vi "Main.vi"(9 "Micro":string, 10 "VISA Com Port":refnum<visa-resource-name>, 11 "Module Admin":refnum<class "Delacor_lib_QMH_Cloneable Module Admin.lvclass">) -> ()   [LabVIEW 2020, in "Serial Device.lvlib"]
doc: "This template is based off of the Queued Message Handler design pattern and the Queued Message Handler project template that ships with LabVIEW.\n\nThe main difference is that the queue is private to this module and communication between modules is performed via Broadcast and Request events.\n\nRequest events are wrapped in public API methods and are handled in the Event Handling Loop (EHL) of this VI. Any module can register for Broadcast events sent by this module. The EHL generates messages based on user interface actions.\n\nThe Message Handling Loop (MHL) processes messages generated by the EHL, or by other messages. The messages are string values, so new messages can be added easily to the Message Cases case structure in the MHL. Each message cluster can also provide an optional value for Message Data, which is a variant that can be converted to whatever message-specific data is required.\n_____\nBased on Delacor QMH Project Template 5.0.0.82."
uses:
  Serial Device.lvlib
  Module Data--cluster.ctl
  <vilib>/Delacor/Delacor QMH/Libraries/Message Queue_class/Delacor_lib_QMH_Message Queue.lvclass
  <vilib>/Delacor/Delacor QMH/Libraries/Message Queue_class/Delacor_lib_QMH_Enqueue Message (Single).vi
  <vilib>/ErrorRing/Error Ring.xnode
  <vilib>/Utility/error.llb/Error Cluster From Error Code.vi
  <vilib>/Delacor/Delacor QMH/Libraries/Cloneable Module Admin_class/Delacor_lib_QMH_Cloneable Module Admin.lvclass
  Stop Argument--cluster.ctl
  <vilib>/Utility/miscctls.llb/LVPointTypeDef.ctl
  Write Port (Reply Payload)--cluster.ctl
  Write Port Argument--cluster.ctl
  Abstract/Serial Device/Serial Device.lvclass
  Implementation/Simulado/Simulado.lvclass
  Implementation/NXP/NXP.lvclass
  Implementation/Cypress/Cypress.lvclass
  C:/Users/celun/Desktop/FORK/ProyectoFinalIV2020/LectorADC3Micros/Abstract/Serial Device/Serial Device.lvclass
  C:/Users/celun/Desktop/FORK/ProyectoFinalIV2020/LectorADC3Micros/Implementation/Simulado/Simulado.lvclass
  C:/Users/celun/Desktop/FORK/ProyectoFinalIV2020/LectorADC3Micros/Implementation/NXP/NXP.lvclass
  C:/Users/celun/Desktop/FORK/ProyectoFinalIV2020/LectorADC3Micros/Implementation/Cypress/Cypress.lvclass
panel:
  out "Response":string
  in  "Read ADC":bool
  in  "ADC Channel":dbl
  in  "Set Value":bool
  in  "OFF/ON":bool
  in  "Pín":dbl
  in  "Port 2":dbl
  in  "Read Pin":bool
  out "Value":bool
  in  "Pín 2":dbl
  in  "Port 3":dbl
  in  "Set Port":bool
  in  "Value":string
  in  "Port":dbl
  out "Leds":bool[](array[boolean])
  in  "Read Pin 2":bool
  in  "Port 4":dbl
  out "error out":errorcluster
  out "Status":string
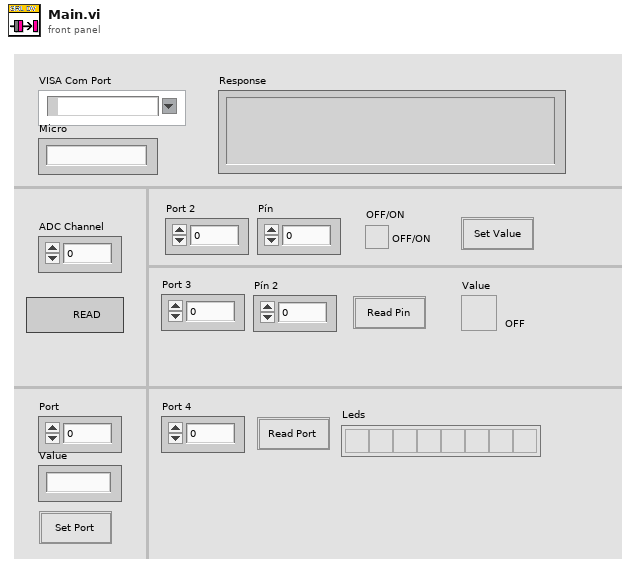
[diagram p1: front panel]
types:
  T1 = typedef "Serial Device.lvlib/Request Events--cluster.ctl" = cluster{"Stop Module":refnum<user-event>, "Show Panel":refnum<user-event>, "Hide Panel":refnum<user-event>, "Show Diagram":refnum<user-event>, "Get Module Execution Status":refnum<user-event>, "Write Port":refnum<user-event>}
  T2 = typedef "Serial Device.lvlib/Module Data--cluster.ctl" = cluster{"Status":string}
  T3 = enum32{"invalid lock state", "Not Locked", "Locked (No Password)", "Password-protected"}
  T4 = typedef "Serial Device.lvlib/Stop Argument--cluster.ctl" = cluster{"Module ID":i32, "Origin":string, "Exit via Stop Module Req?":bool, "Wait for Module to stop?":bool}
  T5 = typedef "Serial Device.lvlib/Write Port Argument--cluster.ctl" = cluster{"Module ID":i32, "Value":string, "Port":dbl, "Wait Notifier":refnum<notifier>, "wait for reply":bool}
  T6 = enum32{"Invalid", "Standard", "Closed", "Hidden", "Minimized", "Maximized"}
  T7 = typedef "LVPointTypeDef.ctl" = cluster{"Horizontal":i16, "Vertical":i16}
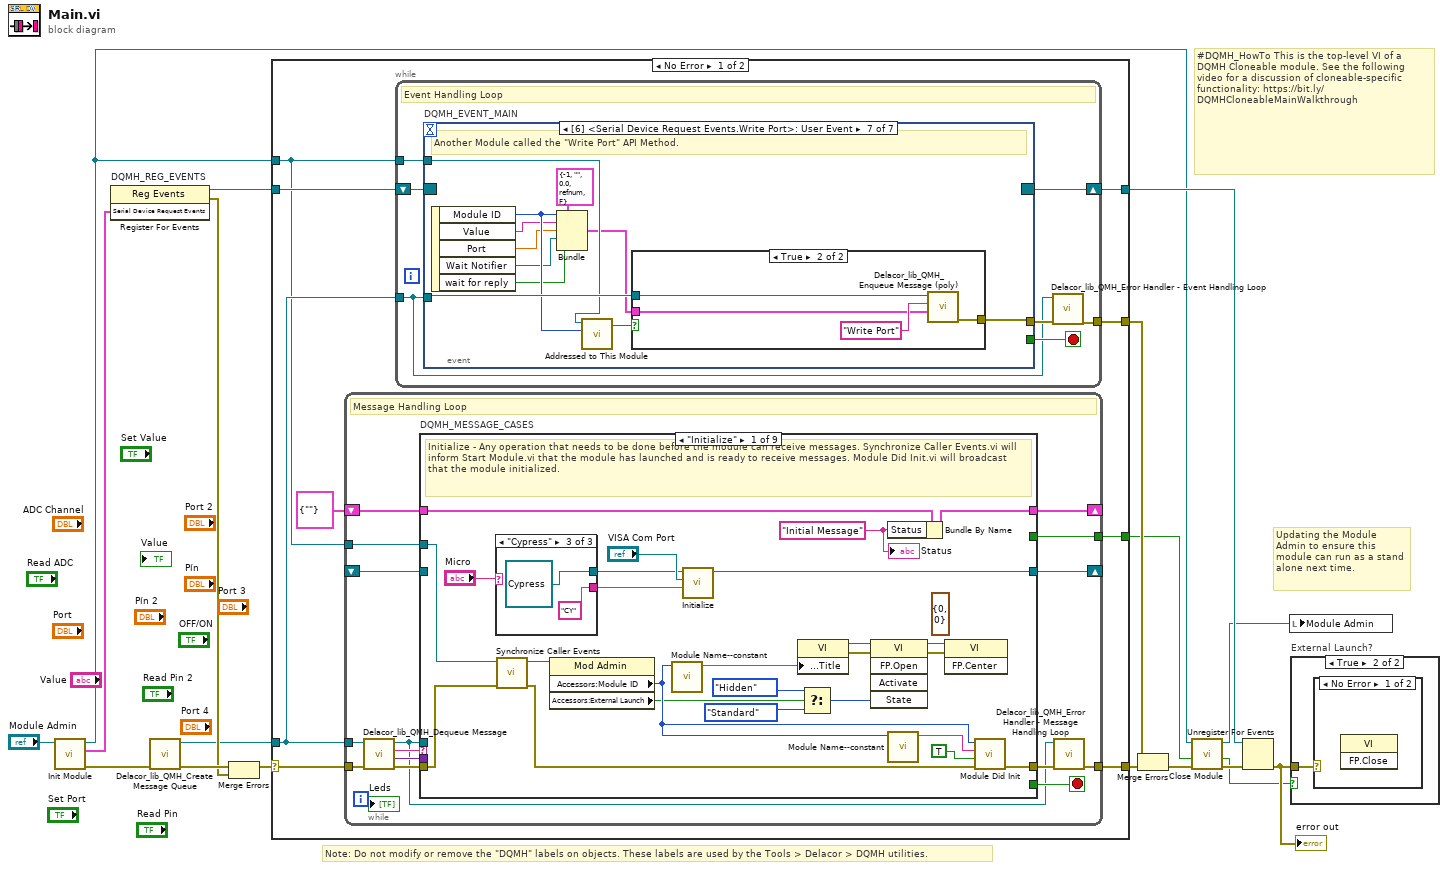
[diagram p0: block diagram]
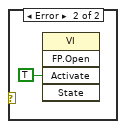
[diagram p3: hidden frame]
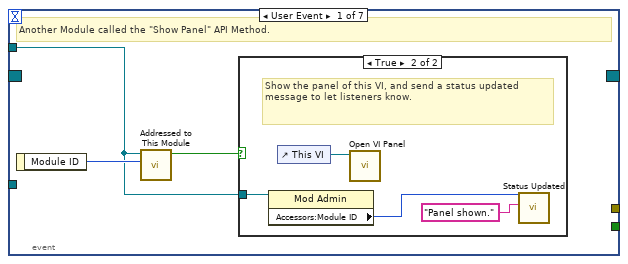
[diagram p4: hidden frame]
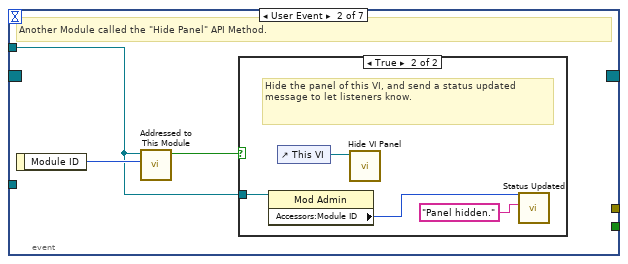
[diagram p6: hidden frame]
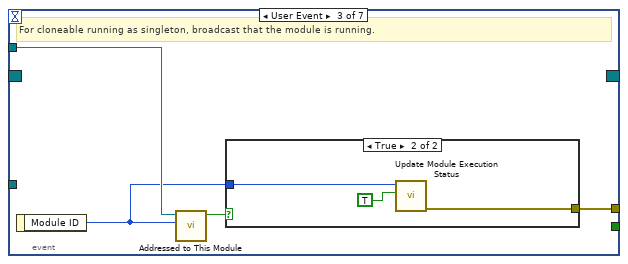
[diagram p8: hidden frame]
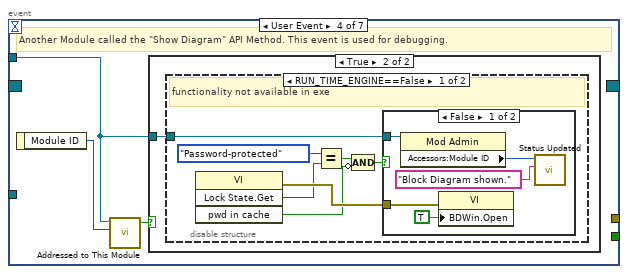
[diagram p10: hidden frame]
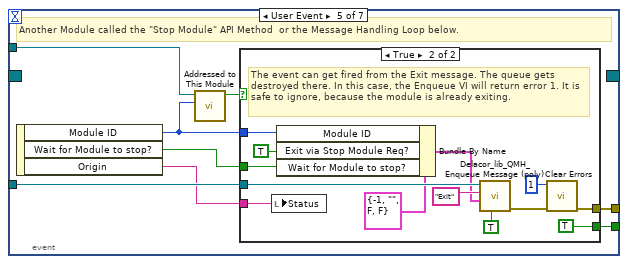
[diagram p14: hidden frame]
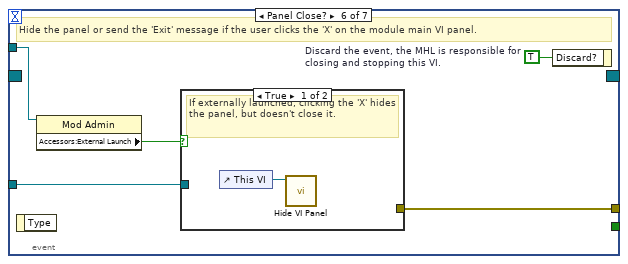
[diagram p16: hidden frame]
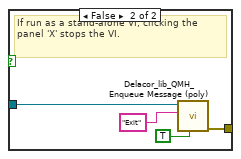
[diagram p17: hidden frame]
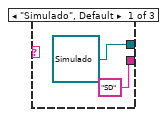
[diagram p19: hidden frame]
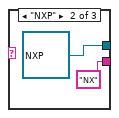
[diagram p20: hidden frame]
diagram:
  # "#DQMH_HowTo This is the top-level VI of a DQMH Cloneable module. See the following video for a discussion of cloneable-specific functionality: https://bit.ly/DQMHCloneableMainWalkthrough"
  # "Note: Do not modify or remove the \"DQMH\" labels on objects. These labels are used by the Tools > Delacor > DQMH utilities."
  # "Updating the Module Admin to ensure this module can run as a stand alone next time."
  n1 = call "Init Module.vi"("Cloneable Module Admin in"="Module Admin") -> ("error out"=w15:errorcluster, "Serial Device Request Events"=w7:T1, "Cloneable Module Admin out"=w4:refnum<class "Delacor_lib_QMH_Cloneable Module Admin.lvclass">)  [unwired: 8 in]
  n2 = register-events "DQMH_REG_EVENTS"(w7) -> (reference out=w8:refnum<event-registration>, error out=w10:errorcluster)  [unwired: 2 in]
  n3 = call <vilib>:"Delacor_lib_QMH_Create Message Queue.vi"("error in (no error)"=w15) -> ("error out"=w12:errorcluster, "Message Queue"=w6:refnum<class "Delacor_lib_QMH_Message Queue.lvclass">)  [unwired: 9 in]
  n4 = Merge Errors(w12, w10) -> (w11:errorcluster)
  n5 = case shown="No Error" w11 {
    selector: w11 -> [w25 w247]
    tunnel: [w27 w246] -> w16
    tunnel: [w24 w254] -> w9
    tunnel: w8 -> [w22 w254]
    tunnel: w6 -> [w21 w245]
    tunnel: [w26 _] -> w17
    tunnel: w4 -> [w20 w250]
    tunnel: [w19 _] -> w2
    frame No Error {
      n6 = while {
        tunnel: w21 -> [w123]
        shift-right: [w127] -> _
        shift-left: T2 {"Status"=""} ("Data Cluster") -> [w128]
        tunnel: w25 -> [w131]
        tunnel: [w129] -> w27
        tunnel: w20 -> [w121]
        tunnel: [w120] -> w19
        shift-right: [w119] -> _
        shift-left: _ -> [w118]
        stop <- w126 stop-if-true
        # "Message Handling Loop"
        n7 = call-dynamic "Delacor_lib_QMH_Dequeue Message.vi"("error in (no error)"=w131, "Message Queue in"=w123) -> ("error out"=w130:errorcluster, "Message Data"=w124:variant, "Message"=w125:string, "Message Queue out"=w122:refnum<class "Delacor_lib_QMH_Message Queue.lvclass">)  [unwired: 6 in]
        n8 = case "DQMH_MESSAGE_CASES" shown="\"Initialize\"" w125 {
          selector: w125 -> [_ _ _ _ _ _ _ _ w232]
          tunnel: w122 -> [_ _ w169 _ _ _ w197 w222 _]
          tunnel: w130 -> [w155 w165 w182 w189 w192 w194 w206 w228 w234]
          tunnel: [w153 w165 w177 w187 w191 w194 w202 w225 w235] -> w132
          tunnel: w128 -> [w146 w164 w181 w188 w190 w193 w201 w221 w233]
          tunnel: [w145 w164 w181 w188 w190 w193 w201 w221 w233] -> w127
          tunnel: [_ _ _ _ _ _ _ w220 _] -> w126
          tunnel: w124 -> [_ _ w180 w186 _ _ w200 w218 _]
          tunnel: w121 -> [w140 _ _ _ _ _ w199 w214 w230]
          tunnel: [_ _ _ _ _ _ _ w216 _] -> w120
          tunnel: [w136 _ w170 w183 _ _ _ _ _] -> w119
          tunnel: w118 -> [_ _ w175 w183 _ _ _ _ _]
          frame "Initialize" {
            (unwired) T7 {"Horizontal"=0, "Vertical"=0} ("Origin")
            w138 = "Initial Message" ("Initial Message")
            # "Initialize - Any operation that needs to be done before the module can receive messages. Synchronize Caller Events.vi will inform Start Module.vi that the module has launched and is ready to receive messages. Module Did Init.vi will broadcast that the module initialized."
            n9 = case shown="\"Cypress\"" "Micro" {
              tunnel: [refnum<class "Simulado.lvclass"> refnum ("Simulado.lvclass") refnum<class "NXP.lvclass"> refnum ("NXP.lvclass") refnum<class "Cypress.lvclass"> refnum ("Cypress.lvclass")] -> w134
              tunnel: ["SD" "NX" "CY"] -> w133
              frame "Simulado", Default {
              }
              frame "NXP" {
              }
              frame "Cypress" {
              }
            }
            n10 = call "Synchronize Caller Events.vi"("error in (no error)"=w155, "Module Admin"=w140) -> ("error out"=w154:errorcluster, "Module Admin out"=w139:refnum<class "Delacor_lib_QMH_Cloneable Module Admin.lvclass">)  [unwired: 8 in]
            n11 = property class="Mod Admin"(reference=w139) -> ("Accessors:Module ID"=w142:i32, "Accessors:External Launch"=w141:bool)  [unwired: 1 in, 2 out]
            n12 = call "Module Name--constant.vi"("Module ID"=w142) -> ("Module Name"=w150:string)  [unwired: 10 in]
            n13 = call-dynamic "Initialize.vi"("Device"=w133, "VISA Com Port"="VISA Com Port", "Serial Device in"=w134) -> ("Serial Device out"=w136:refnum<class "Serial Device.lvclass">)  [unwired: 7 in, 1 out]
            n14 = property class="VI"("Front Panel.Title"=w150) -> (reference out=w152:refnum<vi>, error out=w157:errorcluster)  [unwired: 2 in]
            n15 = Select(t=T6."Hidden" ("State"), s=w141, f=T6."Standard" ("State")) -> (s? t:f=w147:T6)
            n16 = invoke class="VI" method="FP.Open"(reference=w152, error in=w157, "State"=w147) -> (reference out=w151:refnum<vi>, error out=w156:errorcluster)  [unwired: 2 in, 3 out]
            n17 = Bundle By Name(cluster=w146, "Status"=w138) -> (w145:T2)
            n18 = call "Module Name--constant.vi"("Module ID"=w142) -> ("Module Name"=w143:string)  [unwired: 10 in]
            n19 = invoke class="VI" method="FP.Center"(reference=w151, error in=w156) -> ()  [unwired: 1 in, 3 out]
            n20 = call "Module Did Init.vi"("error in (no error)"=w154, "Initialized?"=TRUE, "Origin"=w143, "Module ID"=w142) -> ("error out"=w153:errorcluster)  [unwired: 7 in]
            "Status" <- w138
          }
          frame "--- Module Specific ---" {
            # "Separator -- The following cases handle messages specific to this Module."
          }
          frame "Write Port" {
            # "Evento para escribir en los puertos del micro seleccionado."
            n21 = Variant To Data(error in=w182, type=T5 {"Module ID"=-1, "Value"="", "Port"=0.0, "Wait Notifier"=refnum, "wait for reply"=FALSE} ("Write Port Argument"), Variant=w180) -> (data=w178:T5, error out=w176:errorcluster)
            n22 = Unbundle By Name(w178) -> ("Port"=w174:dbl, "Value"=w173:string)
            n23 = call-dynamic "WritePortStatus.vi"("error in (no error)"=w176, "Value"=w173, "Port"=w174, "Serial Device in"=w175) -> ("error out"=w171:errorcluster, "Serial Device out"=w172:refnum<class "Serial Device.lvclass">)  [unwired: 6 in]
            n24 = call-dynamic "ReadCommand.vi"("error in (no error)"=w171, "Serial Device in"=w172) -> ("error out"=w166:errorcluster, "Read buffer"=w167:string, "Serial Device out"=w170:refnum<class "Serial Device.lvclass">)  [unwired: 7 in]
            n25 = call-poly <vilib>:"Delacor_lib_QMH_Enqueue Message (poly).vi"("error in (no error)"=w166, "Message Data"=w167, "Message"="RespuestaMicro", "Message Queue in"=w169) -> ("error out"=w177:errorcluster)  [unwired: 6 in, 1 out]
          }
          frame "RespuestaMicro" {
            n26 = Variant To Data(error in=w189, type="", Variant=w186) -> (data=→"Response":string, error out=w187:errorcluster)
          }
          frame "---Copy This Frame---" {
            # "Duplicate this frame when creating new messages.  Change this comment in the duplicated frame to describe this message."
            n27 = Merge Errors(w192) -> (w191:errorcluster)
          }
          frame "--- Exit and Error Handling---" {
            # "Separator - the following cases handle errors and exit messages."
          }
          frame "Error" {
            # "#CodeRecommended - If you ever change the name of this \"Error\" message, you'll need to update the name in the Check Loop Error.vi as well."
            # "#CodeRecommended - If the module is running in standalone mode (External Launch = FALSE), this code will pop up an error dialog and call the 'Exit' message if an error occurs. Add more fine-grained error handling here."
            # "Error - Check the error message data and respond accordingly. This message is sent by the \"Error Handler\" VIs at the end of each loop in this application."
            n28 = property class="Mod Admin"(reference=w199) -> ("Accessors:External Launch"=w198:bool, "Accessors:Module ID"=w195:i32)  [unwired: 1 in, 2 out]
            n29 = Variant To Data(error in=w206, type=errorcluster {"status"=FALSE, "code"=0, "source"=""} ("error constant"), Variant=w200) -> (data=w207:errorcluster, error out=w204:errorcluster)
            n30 = call "Module Name--constant.vi"("Module ID"=w195) -> ("Module Name"=w196:string)  [unwired: 10 in]
            n31 = call "Error Reported.vi"("Additional Information"=w196, "Error"=w207, "Module ID"=w195) -> ()  [unwired: 8 in, 1 out]
            n32 = case shown="False" w198 {
              tunnel: [w212 _] -> w203
              tunnel: w197 -> [w210 _]
              tunnel: w207 -> [w211 _]
              frame False {
                # "If the module is running standalone, then pop up an error dialog and call the \"Exit\" message."
                n33 = call <vilib>:"Simple Error Handler.vi"("error in (no error)"=w211) -> ()  [unwired: 4 in, 5 out]
                n34 = call-poly <vilib>:"Delacor_lib_QMH_Enqueue Message (poly).vi"("Priority Message? (F)"=TRUE, "Message"="Exit", "Message Queue in"=w210) -> ("error out"=w212:errorcluster)  [unwired: 7 in, 1 out]
              }
              frame True {
                # "If the module was launched externally, calling the Error Reported broadcast VI is the only action performed by the \"Error\" message. The module's caller can then process the error appropriately."
              }
            }
            n35 = Merge Errors(w204, w203) -> (w202:errorcluster)
            n36 = local write "error out"(w202) -> ()
          }
          frame "Exit" {
            w219 = 91  # 91: not all Exit messages will have an argument
            w220 = TRUE  # Stop the VI
            # "Release the message queue reference"
            # "#CodeNeeded - Add any required cleanup code here."
            # "Exit - Exit the application."
            n37 = Variant To Data(error in=w228, type=T4 {"Module ID"=-1, "Origin"="", "Exit via Stop Module Req?"=FALSE, "Wait for Module to stop?"=FALSE} ("Stop Argument"), Variant=w218) -> (data=w215:T4, error out=w223:errorcluster)
            n38 = call <vilib>:"Clear Errors.vi"("error in (no error)"=w223, "specific error code to clear (0: all)"=w219) -> ("error out"=w227:errorcluster)  [unwired: 4 in, 1 out]
            n39 = control-ref of="This VI"() -> (w213:refnum<vi>)
            n40 = call-dynamic "Delacor_lib_QMH_Release Message Queue.vi"("error in (no error)"=w227, "Message Queue"=w222) -> ("error out"=w226:errorcluster)  [unwired: 9 in]
            n41 = call "Handle Exit.vi"("Stop Argument"=w215, "Module Admin in"=w214, "VI reference"=w213) -> ("error out"=w224:errorcluster, "Wait for Stop?"=w216:bool)  [unwired: 7 in]
            n42 = Merge Errors(w226, w224) -> (w225:errorcluster)
          }
          frame Default {
            # "'Default' case only runs if there is a message that isn't defined in any of the other cases.  Output a programming error."
            n43 = property class="Mod Admin"(reference=w230) -> ("Accessors:Module ID"=w229:i32)  [unwired: 1 in, 2 out]
            n44 = call "Module Name--constant.vi"("Module ID"=w229) -> ("Module Name"=w231:string)  [unwired: 10 in]
            n45 = xnode "Error Ring"("parameter 0"=w232, "parameter 1"=w231) -> ("error out"=w236:errorcluster)
            n46 = Merge Errors(w234, w236) -> (w235:errorcluster)
          }
        }
        n47 = call-dynamic "Delacor_lib_QMH_Error Handler - Message Handling Loop.vi"("error in (no error)"=w132, "Message Queue in"=w122) -> ("dup error in"=w129:errorcluster)  [unwired: 8 in, 1 out]
      }
      n48 = while {
        tunnel: w21 -> [w28]
        shift-right: [w31] -> w24
        shift-left: w22 -> [w32]
        tunnel: [w33] -> w26
        tunnel: w20 -> [w29]
        stop <- w30 stop-if-true
        # "Event Handling Loop"
        n49 = event "DQMH_EVENT_MAIN" shown="[6] <Serial Device Request Events.Write Port>: User Event" {
          selector: w32 -> [_ _ _ _ _ _ _]
          dyn-events: [_ _ _ _ _ _ _] -> w31
          timeout: _ -> [_ _ _ _ _ _ _]
          tunnel: [_ _ _ _ w75 _ _] -> w30
          tunnel: w28 -> [_ _ _ _ w78 w94 w113]
          tunnel: [_ _ w52 _ w79 w97 w103] -> w34
          tunnel: w29 -> [w35 w42 w50 w56 w77 w95 w111]
          event User Event {
            # "Another Module called the \"Show Panel\" API Method."
            n50 = event-data() -> ("Module ID"=w36:i32)  [unwired: 1 in]
            n51 = call "Addressed to This Module.vi"("Module ID from Argument"=w36, "Module Admin"=w35) -> ("Addressed to this instance?"=w37:bool)  [unwired: 8 in, 1 out]
            n52 = case shown="True" w37 {
              tunnel: w35 -> [_ w39]
              frame False {
              }
              frame True {
                # "Show the panel of this VI, and send a status updated message to let listeners know."
                n53 = property class="Mod Admin"(reference=w39) -> ("Accessors:Module ID"=w38:i32)  [unwired: 1 in, 2 out]
                n54 = control-ref of="This VI"() -> (w41:refnum<vi>)
                n55 = call "Open VI Panel.vi"("VI"=w41) -> ()  [unwired: 10 in, 1 out]
                n56 = call "Status Updated.vi"("Status"="Panel shown." ("format string"), "Module ID"=w38) -> ()  [unwired: 9 in, 1 out]
              }
            }
          }
          event User Event {
            # "Another Module called the \"Hide Panel\" API Method."
            n57 = event-data() -> ("Module ID"=w43:i32)  [unwired: 1 in]
            n58 = call "Addressed to This Module.vi"("Module ID from Argument"=w43, "Module Admin"=w42) -> ("Addressed to this instance?"=w44:bool)  [unwired: 8 in, 1 out]
            n59 = case shown="True" w44 {
              tunnel: w42 -> [_ w46]
              frame False {
              }
              frame True {
                # "Hide the panel of this VI, and send a status updated message to let listeners know."
                n60 = property class="Mod Admin"(reference=w46) -> ("Accessors:Module ID"=w45:i32)  [unwired: 1 in, 2 out]
                n61 = control-ref of="This VI"() -> (w48:refnum<vi>)
                n62 = call "Hide VI Panel.vi"("VI"=w48) -> ()  [unwired: 10 in, 1 out]
                n63 = call "Status Updated.vi"("Status"="Panel hidden." ("format string"), "Module ID"=w45) -> ()  [unwired: 9 in, 1 out]
              }
            }
          }
          event User Event {
            # "For cloneable running as singleton, broadcast that the module is running."
            n64 = event-data() -> ("Module ID"=w49:i32)  [unwired: 1 in]
            n65 = call "Addressed to This Module.vi"("Module ID from Argument"=w49, "Module Admin"=w50) -> ("Addressed to this instance?"=w51:bool)  [unwired: 8 in, 1 out]
            n66 = case shown="True" w51 {
              tunnel: [_ w55] -> w52
              tunnel: w49 -> [_ w54]
              frame False {
              }
              frame True {
                n67 = call "Update Module Execution Status.vi"("Running?"=TRUE, "Module ID"=w54) -> ("error out"=w55:errorcluster)  [unwired: 9 in]
              }
            }
          }
          event User Event {
            # "Another Module called the \"Show Diagram\" API Method. This event is used for debugging."
            n68 = event-data() -> ("Module ID"=w57:i32)  [unwired: 1 in]
            n69 = call "Addressed to This Module.vi"("Module ID from Argument"=w57, "Module Admin"=w56) -> ("Addressed to this instance?"=w58:bool)  [unwired: 8 in, 1 out]
            n70 = case shown="True" w58 {
              tunnel: w56 -> [_ w59]
              frame False {
              }
              frame True {
                n71 = disable-structure shown="RUN_TIME_ENGINE==False" {
                  disable-tunnel: w59 -> [w60 _]
                  frame condition #0 (active) {
                    # "functionality not available in exe"
                    n72 = invoke class="VI" method="Lock State.Get"() -> (error out=w66:errorcluster, "Get Lock State"=w65:T3, "pwd in cache"=w62:bool)  [unwired: 4 in, 1 out]
                    n73 = Equal?(x=T3."Password-protected", y=w65) -> (x = y?=w63:bool)
                    n74 = Compound Arithmetic op=AND(w63, invert w62) -> (w61:bool)
                    n75 = case shown="False" w61 {
                      tunnel: w66 -> [w71 _]
                      tunnel: w60 -> [w68 _]
                      frame False {
                        n76 = property class="Mod Admin"(reference=w68) -> ("Accessors:Module ID"=w67:i32)  [unwired: 1 in, 2 out]
                        n77 = property class="VI"(error in=w71, "BDWin.Open"=TRUE ("Block Diagram Window:Open")) -> ()  [unwired: 1 in, 2 out]
                        n78 = call "Status Updated.vi"("Status"="Block Diagram shown." ("format string"), "Module ID"=w67) -> ()  [unwired: 9 in, 1 out]
                      }
                      frame True {
                        # "Password-protected VI, and the password is not in the cache. Do not show the diagram."
                      }
                    }
                  }
                  frame condition #1 {
                  }
                }
              }
            }
          }
          event User Event {
            # "Another Module called the \"Stop Module\" API Method  or the Message Handling Loop below."
            n79 = event-data() -> ("Module ID"=w73:i32, "Wait for Module to stop?"=w74:bool, "Origin"=w72:string)  [unwired: 1 in]
            n80 = call "Addressed to This Module.vi"("Module ID from Argument"=w73, "Module Admin"=w77) -> ("Addressed to this instance?"=w76:bool)  [unwired: 8 in, 1 out]
            n81 = case shown="True" w76 {
              tunnel: [_ w91] -> w79
              tunnel: w78 -> [_ w87]
              tunnel: [_ TRUE] -> w75
              tunnel: w74 -> [_ w82]
              tunnel: w73 -> [_ w84]
              tunnel: w72 -> [_ w80]
              frame False {
              }
              frame True {
                # "The event can get fired from the Exit message. The queue gets destroyed there. In this case, the Enqueue VI will return error 1. It is safe to ignore, because the module is already exiting."
                n82 = local write "Status"(w80) -> ()
                n83 = Bundle By Name(cluster=T4 {"Module ID"=-1, "Origin"="", "Exit via Stop Module Req?"=FALSE, "Wait for Module to stop?"=FALSE} ("Stop Argument"), "Module ID"=w84, "Exit via Stop Module Req?"=TRUE, "Wait for Module to stop?"=w82) -> (w81:T4)
                n84 = call-poly <vilib>:"Delacor_lib_QMH_Enqueue Message (poly).vi"("Priority Message? (F)"=TRUE, "Message Data"=w81, "Message"="Exit", "Message Queue in"=w87) -> ("error out"=w92:errorcluster)  [unwired: 6 in, 1 out]
                n85 = call <vilib>:"Clear Errors.vi"("error in (no error)"=w92, "specific error code to clear (0: all)"=1) -> ("error out"=w91:errorcluster)  [unwired: 4 in, 1 out]
              }
            }
          }
          event Panel Close? {
            w96 = TRUE  # Discard the event, the MHL is responsible for closing and stopping this VI.
            # "Hide the panel or send the 'Exit' message if the user clicks the 'X' on the module main VI panel."
            n86 = event-data() -> ()  [unwired: 1 in, 1 out]
            n87 = property class="Mod Admin"(reference=w95) -> ("Accessors:External Launch"=w93:bool)  [unwired: 1 in, 2 out]
            n88 = case shown="True" w93 {
              tunnel: w94 -> [_ w101]
              tunnel: [_ w102] -> w97
              frame True {
                # "If externally launched, clicking the 'X' hides the panel, but doesn't close it."
                n89 = control-ref of="This VI"() -> (w98:refnum<vi>)
                n90 = call "Hide VI Panel.vi"("VI"=w98) -> ()  [unwired: 10 in, 1 out]
              }
              frame False {
                # "If run as a stand-alone VI, clicking the panel 'X' stops the VI."
                n91 = call-poly <vilib>:"Delacor_lib_QMH_Enqueue Message (poly).vi"("Priority Message? (F)"=TRUE, "Message"="Exit", "Message Queue in"=w101) -> ("error out"=w102:errorcluster)  [unwired: 7 in, 1 out]
              }
            }
            n92 = event-data("Discard?"=w96) -> ()  [unwired: 1 in, 1 out]
          }
          event User Event {
            # "Another Module called the \"Write Port\" API Method."
            n93 = event-data() -> ("Module ID"=w108:i32, "Value"=w107:string, "Port"=w106:dbl, "Wait Notifier"=w105:refnum<notifier>, "wait for reply"=w104:bool)  [unwired: 1 in]
            n94 = Bundle(cluster=T5 {"Module ID"=-1, "Value"="", "Port"=0.0, "Wait Notifier"=refnum, "wait for reply"=FALSE} ("Write Port Argument"), "Module ID"=w108, "Value"=w107, "Port"=w106, "Wait Notifier"=w105, "wait for reply"=w104) -> (w109:T5)
            n95 = call "Addressed to This Module.vi"("Module ID from Argument"=w108, "Module Admin"=w111) -> ("Addressed to this instance?"=w112:bool)  [unwired: 8 in, 1 out]
            n96 = case shown="True" w112 {
              tunnel: w113 -> [_ w117]
              tunnel: w109 -> [_ w115]
              tunnel: [_ w114] -> w103
              frame False {
              }
              frame True {
                n97 = call-poly <vilib>:"Delacor_lib_QMH_Enqueue Message (poly).vi"("Message Data"=w115, "Message"="Write Port", "Message Queue in"=w117) -> ("error out"=w114:errorcluster)  [unwired: 7 in, 1 out]
              }
            }
          }
        }
        n98 = call-dynamic "Delacor_lib_QMH_Error Handler - Event Handling Loop.vi"("error in (no error)"=w34, "Message Queue in"=w28) -> ("dup error in"=w33:errorcluster)  [unwired: 8 in, 1 out]
      }
    }
    frame Error {
      n99 = call "Synchronize Caller Events.vi"("Module Admin"=w250) -> ("Module Admin out"=w249:refnum<class "Delacor_lib_QMH_Cloneable Module Admin.lvclass">)  [unwired: 9 in, 1 out]
      n100 = property class="Mod Admin"(reference=w249) -> ("Accessors:Module ID"=w248:i32)  [unwired: 1 in, 2 out]
      n101 = call-dynamic "Delacor_lib_QMH_Release Message Queue.vi"("error in (no error)"=w247, "Message Queue"=w245) -> ("error out"=w246:errorcluster)  [unwired: 9 in]
      n102 = call "Module Name--constant.vi"("Module ID"=w248) -> ("Module Name"=w253:string)  [unwired: 10 in]
      n103 = Format Into String(format string="An error occurred during initialization. %s is no longer running.", w253) -> (resulting string=w251:string)  [unwired: 2 in, 1 out]
      n104 = call "Error Reported.vi"("Additional Information"=w251, "Error"=w246, "Module ID"=w248) -> ()  [unwired: 8 in, 1 out]
    }
  }
  n105 = Merge Errors(w17, w16) -> (w18:errorcluster)
  n106 = call "Close Module.vi"("error in"=w18, "Wait for stop?"=w2, "Module Admin in"=w4) -> ("error out"=w14:errorcluster, "External Launch"=w1:bool, "Module Admin out"=w3:refnum<class "Delacor_lib_QMH_Cloneable Module Admin.lvclass">)  [unwired: 6 in]
  n107 = Unregister For Events(event registration refnum=w9, error in=w14) -> (error out=w13:errorcluster)
  "error out" <- w13
  n108 = local write "Module Admin"(w3) -> ()
  n109 = case "External Launch?" shown="True" w1 {
    tunnel: w13 -> [_ w255]
    frame False {
    }
    frame True {
      n110 = case shown="No Error" w255 {
        frame No Error {
          n111 = invoke class="VI" method="FP.Close"() -> ()  [unwired: 3 in, 3 out]
        }
        frame Error {
          n112 = invoke class="VI" method="FP.Open"("Activate"=TRUE ("Activate?")) -> ()  [unwired: 4 in, 5 out]
        }
      }
    }
  }
